vi "Read System Version.vi"(8 "error in (no error)":errorcluster, 11 "VISA resource name":refnum<visa-resource-name>) -> (0 "error out":errorcluster, 2 "Version":string, 3 "VISA resource name out":refnum<visa-resource-name>)   [LabVIEW 2018, in "LTB-1.lvlib" / "3150.lvlib"]
doc: "Reads the 3150 identification string."
uses:
  3150.lvlib
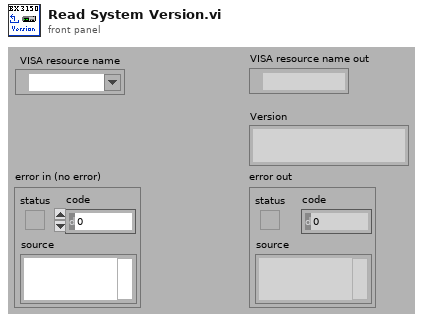
[diagram p1: front panel]
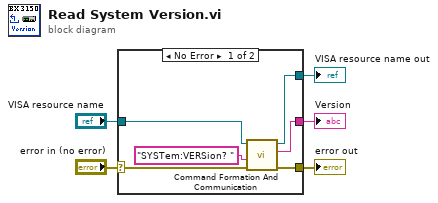
[diagram p0: block diagram]
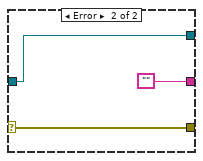
[diagram p2: hidden frame]
diagram:
  n1 = case shown="No Error" "error in (no error)" {
    selector: "error in (no error)" -> [w11 w14]
    tunnel: [w10 w14] -> w5
    tunnel: [w9 w13] -> w2
    tunnel: "VISA resource name" -> [w8 w13]
    tunnel: [w7 ""] -> w1
    frame No Error {
      n2 = call "Command Formation And Communication.vi"("error in (no error)"=w11, "Command"="SYSTem:VERSion? ", "VISA resource name"=w8) -> ("error out"=w10:errorcluster, "Response"=w7:string, "VISA resource name out"=w9:refnum<visa-resource-name>)  [unwired: 2 in, 4 out]
    }
    frame Error {
    }
  }
  "error out" <- w5
  "Version" <- w1
  "VISA resource name out" <- w2
